vi "4Pi Dual DM - Get Save Paths.vi"() -> (4 "Modes Path":path, 8 "DM01 Path":path, 15 "DM02 Path":path)   [LabVIEW 2020]
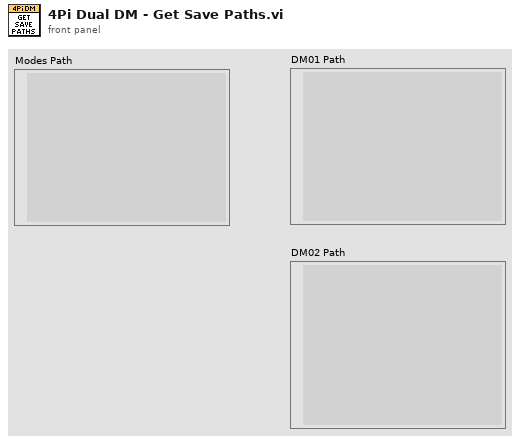
[diagram p1: front panel]
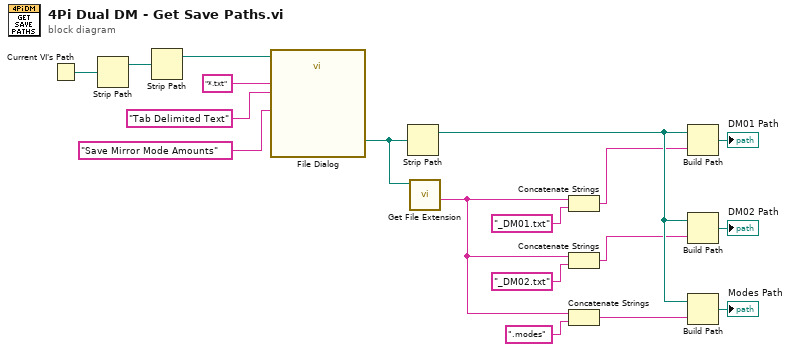
[diagram p0: block diagram]
diagram:
  n1 = Current VI's Path() -> (path=w18:path)
  n2 = Strip Path(path=w18) -> (stripped path=w17:path)  [unwired: 1 out]
  n3 = Strip Path(path=w17) -> (stripped path=w16:path)  [unwired: 1 out]
  n4 = call "File Dialog"("start path"=w16, "prompt"="Save Mirror Mode Amounts", "pattern (all files)"="*.txt", "pattern label"="Tab Delimited Text") -> ("selected path"=w12:path)  [unwired: 8 in, 3 out]
  n5 = Strip Path(path=w12) -> (stripped path=w11:path)  [unwired: 1 out]
  n6 = call <vilib>:"Get File Extension.vi"("file"=w12) -> ("filename without extension"=w10:string)  [unwired: 6 in, 4 out]
  n7 = Concatenate Strings(w10, "_DM01.txt" ("string")) -> (w6:string)
  n8 = Concatenate Strings(w10, "_DM02.txt" ("string")) -> (w5:string)
  n9 = Concatenate Strings(w10, ".modes" ("string")) -> (w4:string)
  n10 = Build Path(base path=w11, name or relative path=w6) -> (appended path=→"DM01 Path":path)
  n11 = Build Path(base path=w11, name or relative path=w5) -> (appended path=→"DM02 Path":path)
  n12 = Build Path(base path=w11, name or relative path=w4) -> (appended path=→"Modes Path":path)
